vi "TB-Update Spectrum Average.vi"(0 "mic":dbl[](array[numeric]), 5 "stim":dbl[](array[numeric]), 7 "state in":T1) -> (4 "RMS":dbl, 6 "Mag":dbl[](array[numeric]), 8 "state out":T1)   [LabVIEW 2020]
uses:
  Typedefs/TB-Runtime state.ctl
  <vilib>/sound2/lvsound2.llb/Sound File Refnum.ctl
  Typedefs/TB-Setup Log.ctl
  Typedefs/TB-Analysis State.ctl
  7a50cbd8-b61d-4096-9ff7-3cd3d19ac463.vi
  <vilib>/Analysis/2dsp.llb/Cross Power (DBL).vi
  540905a8-cfc6-4a5d-920d-409e0d5b90c0.vi
  d3894746-8d97-4418-9a34-6a89e30bf3d7.vi
  <vilib>/Analysis/baseanly.llb/Mean.vi
  <vilib>/Analysis/baseanly.llb/Mean (DBL).vi
  epl-vi-lib/Utility VIs/Math VIs/FFT x(t) to dB,Degrees (1D).vi
  <vilib>/Analysis/NI_AALPro.lvlib
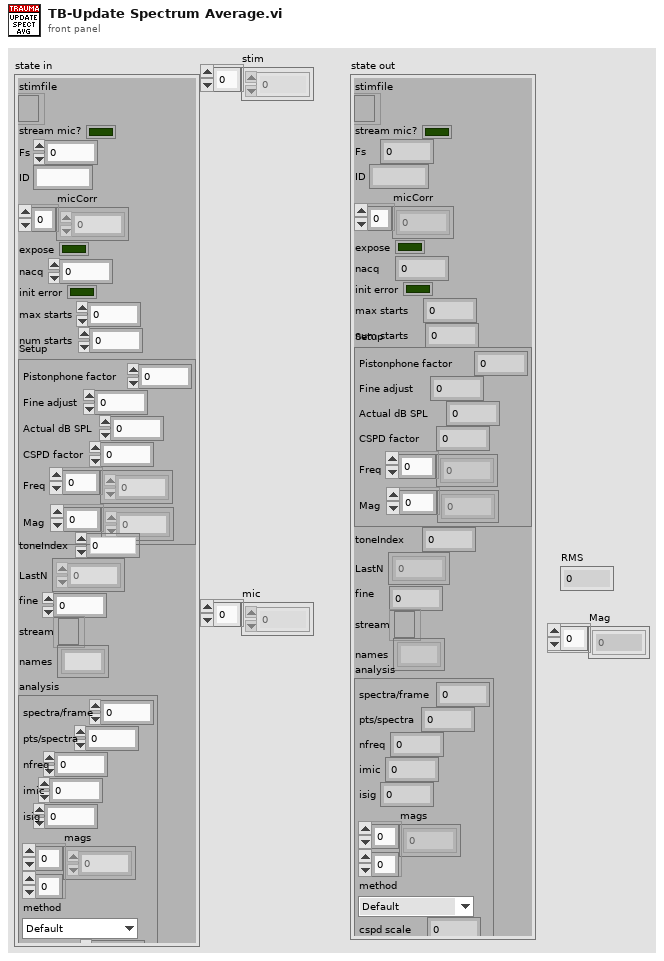
[diagram p1: front panel]
types:
  T1 = typedef "TB-Runtime state.ctl" = cluster{"stimfile":T2, "stream mic?":bool, "Fs":dbl, "ID":string, "micCorr":dbl[], "expose":bool, "nacq":i32, "init error":bool, "max starts":i32, "num starts":i32, "Setup":T3, "toneIndex":i32, "LastN":dbl[], "fine":dbl, "stream":refnum<file>, "names":string[], "analysis":T4}
  T2 = typedef "Sound File Refnum.ctl" = refnum<file>
  T3 = typedef "TB-Setup Log.ctl" = cluster{"Pistonphone factor":dbl, "Fine adjust":dbl, "Actual dB SPL":dbl, "CSPD factor":dbl, "Freq":dbl[], "Mag":dbl[]}
  T4 = typedef "TB-Analysis State.ctl" = cluster{"spectra/frame":i32, "pts/spectra":i32, "nfreq":i32, "imic":i32, "isig":i32, "mags":dbl[][], "method":enum16{"Default", "Periodogram", "Cross-spectrum"}, "cspd scale":dbl}
  T5 = enum16{"Default", "Periodogram", "Cross-spectrum"}
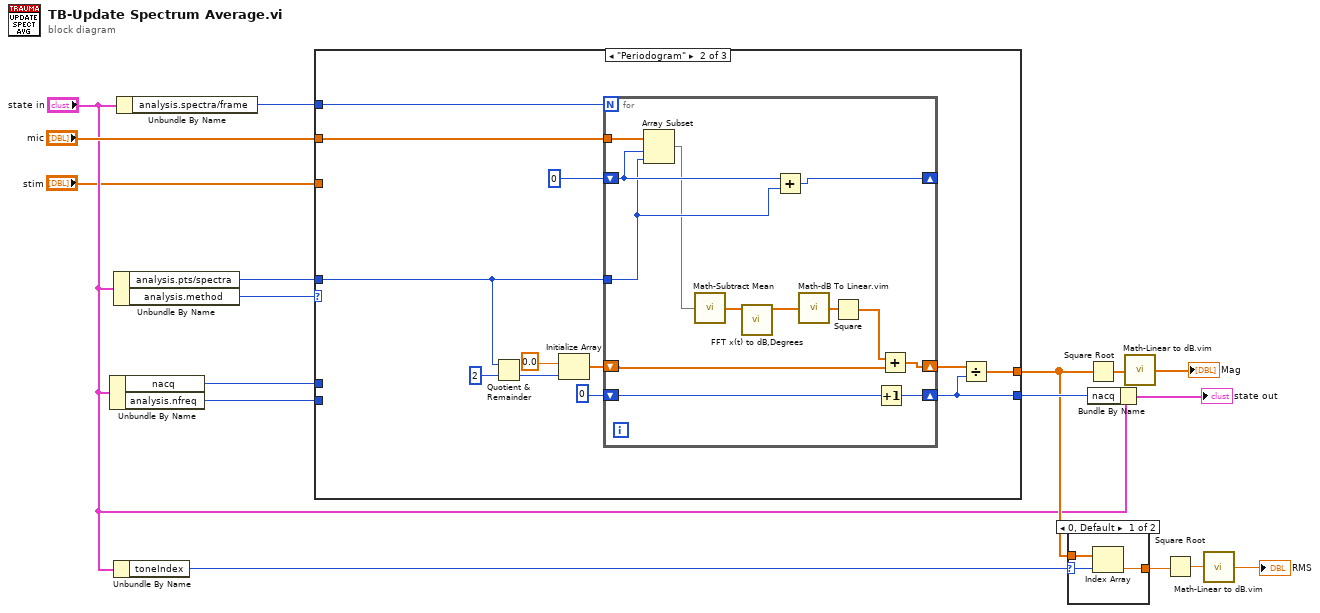
[diagram p0: block diagram]
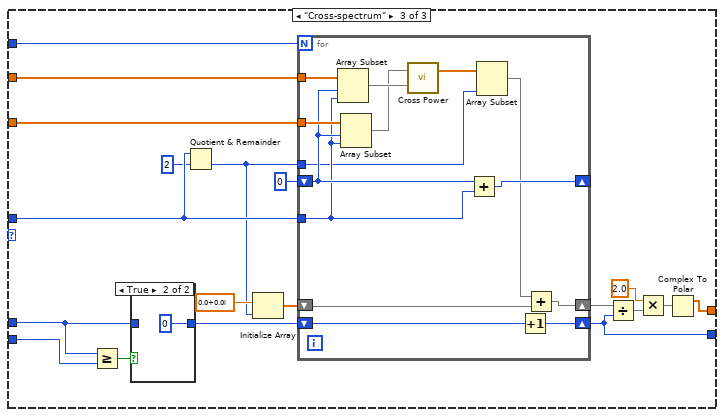
[diagram p3: hidden frame]
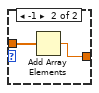
[diagram p5: hidden frame]
diagram:
  n1 = Unbundle By Name("state in") -> ("nacq"=w17:i32, "analysis.nfreq"=w12:i32)
  n2 = Unbundle By Name("state in") -> ("analysis.pts/spectra"=w4:i32, "analysis.method"=w2:T5)
  n3 = Unbundle By Name("state in") -> ("toneIndex"=w6:i32)
  n4 = Unbundle By Name("state in") -> ("analysis.spectra/frame"=w13:i32)
  n5 = case shown="\"Periodogram\"" w2 {
    tunnel: w17 -> [_ _ w61]
    tunnel: w13 -> [_ w28 w58]
    tunnel: w12 -> [_ _ w57]
    tunnel: [_ w27 w56] -> w11
    tunnel: "mic" -> [_ w25 w54]
    tunnel: [_ w24 w47] -> w7
    tunnel: w4 -> [_ w19 w49]
    tunnel: "stim" -> [_ _ w50]
    frame "Default", Default {
    }
    frame "Periodogram" {
      n6 = Quotient & Remainder(x=w19, y=2) -> (floor(x/y)=w18:i32)  [unwired: 1 out]
      n7 = Initialize Array(0.0 ("element"), w18) -> (w22:dbl[])
      n8 = for {
        N: w28 -> [_]
        tunnel: w25 -> [w42]
        shift-right: [w39] -> _
        shift-left: 0 -> [w41]
        tunnel: w19 -> [w40]
        shift-right: [w37] -> w27
        shift-left: 0 -> [w38]
        shift-right: [w35] -> w26
        shift-left: w22 -> [w36]
        n9 = Array Subset(array=w42, index=w41, length=w40) -> (w34:dbl[])
        n10 = call "Math-Subtract Mean.vi"("Y"=w34) -> ("Y - mean(Y)"=w31:dbl[])  [unwired: 4 in]
        n11 = call-poly "FFT x(t) to dB,Degrees.vi"("X"=w31) -> ("+Freq. Mag of FFT (dB rms)"=w30:dbl[])  [unwired: 8 in, 2 out]
        n12 = Add(x=w41, y=w40) -> (x+y=w39:i32)
        n13 = call "Math-dB To Linear.vim"("dB"=w30) -> ("linear"=w33:dbl[])
        n14 = Square(x=w33) -> (x^2=w32:dbl[])
        n15 = Increment(x=w38) -> (x+1=w37:i32)
        n16 = Add(x=w32, y=w36) -> (x+y=w35:dbl[])
      }
      n17 = Divide(x=w26, y=w27) -> (x/y=w24:dbl[])
    }
    frame "Cross-spectrum" {
      n18 = Greater Or Equal?(x=w61, y=w57) -> (x >= y?=w52:bool)
      n19 = case shown="True" w52 {
        tunnel: w61 -> [w76 _]
        tunnel: [w76 0] -> w59
        frame False {
        }
        frame True {
        }
      }
      n20 = Quotient & Remainder(x=w49, y=2) -> (floor(x/y)=w43:i32)  [unwired: 1 out]
      n21 = Initialize Array(cdb 0.0+0.0i ("element"), w43) -> (w51:cdb[])
      n22 = for {
        N: w58 -> [_]
        tunnel: w54 -> [w75]
        shift-right: [w74] -> _
        shift-left: 0 -> [w68]
        tunnel: w49 -> [w67]
        shift-right: [w72] -> w56
        shift-left: w59 -> [w73]
        shift-right: [w70] -> w55
        shift-left: w51 -> [w71]
        tunnel: w50 -> [w69]
        tunnel: w43 -> [w63]
        n23 = Array Subset(array=w75, index=w68, length=w67) -> (w66:dbl[])
        n24 = Array Subset(array=w69, index=w68, length=w67) -> (w65:dbl[])
        n25 = call-poly <vilib>:"Cross Power.vi"("Y"=w66, "X"=w65) -> ("Sxy"=w64:cdb[])  [unwired: 1 out]
        n26 = Add(x=w68, y=w67) -> (x+y=w74:i32)
        n27 = Array Subset(array=w64, length=w63) -> (w62:cdb[])  [unwired: 1 in]
        n28 = Increment(x=w73) -> (x+1=w72:i32)
        n29 = Add(x=w62, y=w71) -> (x+y=w70:cdb[])
      }
      n30 = Divide(x=w55, y=w56) -> (x/y=w45:cdb[])
      n31 = Multiply(x=2.0, y=w45) -> (x*y=w44:cdb[])
      n32 = Complex To Polar(r * e^(i*theta)=w44) -> (r=w47:dbl[])  [unwired: 1 out]
    }
  }
  n33 = case shown="0, Default" w6 {
    selector: w6 -> [w80 _]
    tunnel: [w78 w82] -> w5
    tunnel: w7 -> [w79 w81]
    frame 0, Default {
      n34 = Index Array(array=w79, index=w80) -> (element=w78:dbl)
    }
    frame -1 {
      n35 = Add Array Elements(numeric array=w81) -> (sum=w82:dbl)
    }
  }
  n36 = Square Root(x=w7) -> (sqrt(x)=w10:dbl[])
  n37 = Bundle By Name(cluster="state in", "nacq"=w11) -> (→"state out":T1)
  n38 = call "Math-Linear to dB.vim"("linear"=w10) -> ("dB"=→"Mag":dbl[])
  n39 = Square Root(x=w5) -> (sqrt(x)=w15:dbl)
  n40 = call "Math-Linear to dB.vim"("linear"=w15) -> ("dB"=→"RMS":dbl)
